vi "Telnet Play Script.vi"(8 "error in (no error)":errorcluster, 9 "timeout ms (25000)":i32=25000, 10 "script":cluster{"prompt":string, "reply":string}[](array[cluster]), 11 "telnet connection":T1) -> (0 "error out":errorcluster, 2 "prompts":string[](array[string]), 3 "telnet connection out":T1)   [LabVIEW 2011]
doc: "Executes script on a connection opened with Open Telnet Connection.\n\nThe script consists of entries {prompt, reply}. For each entry the VI reads from the connection until entry.prompt matches the characters read. Then the VI writes the entry.reply to the connection.\n\nThe VI returns the data read from the connection in the prompts array.\n\nThis VI is useful when it is known what data is comming from the connection. For example, you could logon to a UNIX shell (whose prompt character is '%'), execute a command and logout with the script:\n prompt: \"login:\"\n reply: \"<user name>\\r\\n\"\n prompt: \"sword:\"\n reply: \"<user password>\\r\\n\"\n prompt: \"%\"\n reply: \"<command>\\r\\n\"\n prompt: \"%\"\n reply: \"logout\\r\\n\""
uses:
  Telnet Session.ctl
panel:
  out "prompt":string
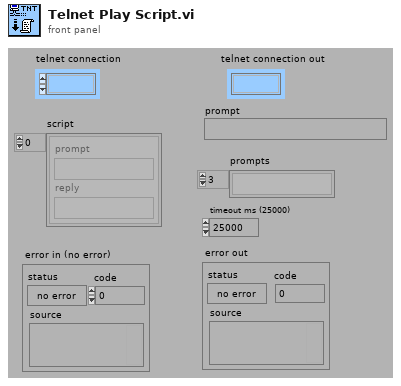
[diagram p1: front panel]
types:
  T1 = typedef "Telnet Session.ctl" = refnum<k1>
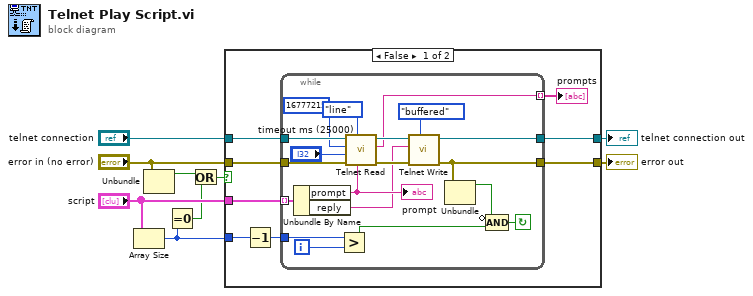
[diagram p0: block diagram]
diagram:
  n1 = Array Size(array="script") -> (size(s)=w4:i32)
  n2 = Unbundle("error in (no error)") -> ("status"=w2:bool)  [unwired: 2 out]
  n3 = Equal To 0?(x=w4) -> (x = 0?=w3:bool)
  n4 = Or(x=w2, y=w3) -> (x .or. y?=w1:bool)
  n5 = case shown="False" w1 {
    tunnel: w4 -> [w16 _]
    tunnel: "script" -> [w15 _]
    tunnel: "telnet connection" -> [w14 w38]
    tunnel: [w13 w38] -> w8
    tunnel: [w12 w37] -> w9
    tunnel: "error in (no error)" -> [w11 w37]
    frame False {
      n6 = Decrement(x=w16) -> (x-1=w17:i32)
      n7 = while {
        tunnel: w14 -> [w36]
        tunnel: [w35] -> w13
        tunnel: [w24] -> w12
        tunnel: w11 -> [w34]
        tunnel: w15 -> [w31] mode=indexing
        tunnel: w17 -> [w25]
        tunnel: [w20] -> w10 mode=indexing
        i -> [w26]
        stop <- w21 continue-if-true
        n8 = Unbundle By Name(w31) -> ("prompt"=w30:string, "reply"=w29:string)
        "prompt" <- w30
        n9 = Greater?(x=w25, y=w26) -> (0:w23:bool)
        n10 = call "Telnet Read.vi"("line separator"=w30, "read mode (normal)"=enum16{"normal", "line", "buffered"}."line", "error in (no error)"=w34, "timeout ms (25000)"="timeout ms (25000)", "bytes to read"=16777215, "telnet connection"=w36) -> ("error out"=w33:errorcluster, "data out"=w20:string, "telnet connection out"=w32:T1)  [unwired: 1 in]
        n11 = call "Telnet Write.vi"("write mode (normal)"=enum16{"normal", "line", "buffered"}."buffered", "error in (no error)"=w33, "data in"=w29, "telnet connection"=w32) -> ("error out"=w24:errorcluster, "telnet  connection out"=w35:T1)  [unwired: 3 in, 1 out]
        n12 = Unbundle(w24) -> ("status"=w22:bool)  [unwired: 2 out]
        n13 = Compound Arithmetic op=AND(invert w22, w23) -> (w21:bool)
      }
      "prompts" <- w10
    }
    frame True {
    }
  }
  "telnet connection out" <- w8
  "error out" <- w9
